vi "Link Control References.vi"(8 "error in (no error)":errorcluster, 10 "Control Map":T1[](array[typedef]), 11 "FunctionGenerator in":refnum<class "FunctionGenerator.lvclass">) -> (0 "error out":errorcluster, 3 "FunctionGenerator out":refnum<class "FunctionGenerator.lvclass">)   [LabVIEW 2019, in "FunctionGenerator.lvlib" / "FunctionGenerator.lvclass"]
uses:
  Library/FunctionGenerator.lvclass
  builds/Instruments/Instruments.lvlibp/Custom Controls/Control Element.ctl
  Library/FunctionGenerator.lvclass/FunctionGenerator.ctl
  builds/Instruments/Instruments.lvlibp/Library/Instruments.lvclass
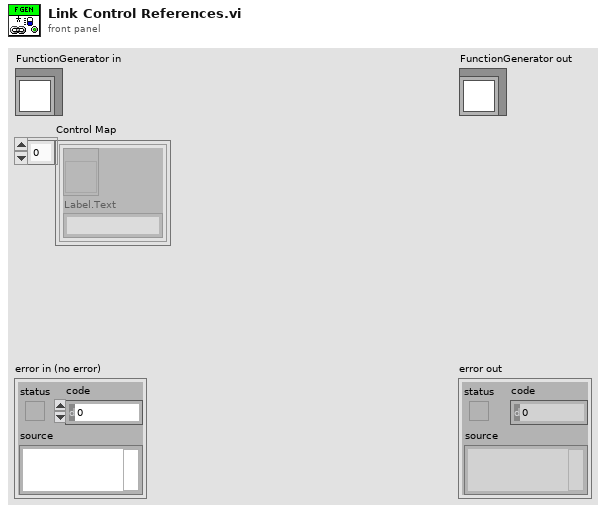
[diagram p1: front panel]
types:
  T1 = typedef "Instruments.lvlibp/Instruments.lvclass/Control Element.ctl" = cluster{refnum<vi>, "Label.Text":string}
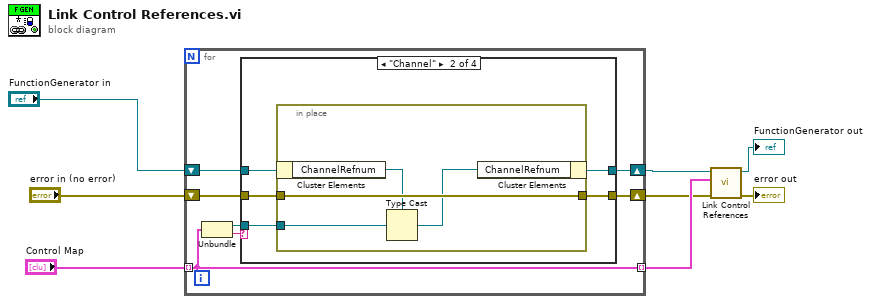
[diagram p0: block diagram]
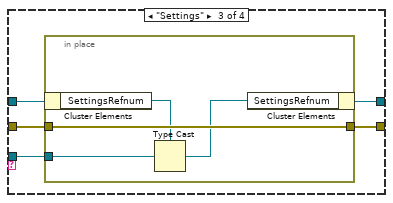
[diagram p3: hidden frame]
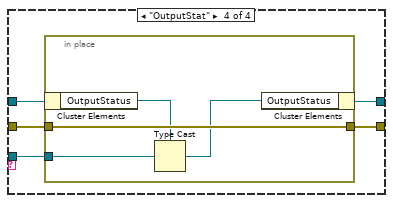
[diagram p4: hidden frame]
diagram:
  n1 = for {
    tunnel: "Control Map" -> [w13] mode=indexing
    tunnel: [w13] -> w5 mode=indexing
    shift-right: [w10] -> w3
    shift-left: "FunctionGenerator in" -> [w14]
    shift-right: [w9] -> w1
    shift-left: "error in (no error)" -> [w15]
    n2 = Unbundle(w13) -> (w11:refnum<vi>, "Label.Text"=w12:string)
    n3 = case shown="\"Channel\"" w12 {
      tunnel: w15 -> [w16 w20 w29 w38]
      tunnel: w14 -> [w17 w22 w31 w40]
      tunnel: w11 -> [_ w18 w27 w36]
      tunnel: [w17 w21 w30 w39] -> w10
      tunnel: [w16 w19 w28 w37] -> w9
      frame Default {
      }
      frame "Channel" {
        n4 = in-place {
          in-place-border: w20 -> [w26]
          in-place-border: [w26] -> w19
          in-place-border: w18 -> [w24]
          n5 = in-place-cluster #1(w22) -> ("ChannelRefnum"=w25:refnum<vi>)
          n6 = Type Cast(type=w25, x=w24) -> (*(type *) &x=w23:refnum<vi>)
          n7 = in-place-cluster #1("ChannelRefnum"=w23) -> (w21:refnum<class "FunctionGenerator.lvclass">)
        }
      }
      frame "Settings" {
        n8 = in-place {
          in-place-border: w29 -> [w35]
          in-place-border: [w35] -> w28
          in-place-border: w27 -> [w33]
          n9 = in-place-cluster #2(w31) -> ("SettingsRefnum"=w34:refnum<vi>)
          n10 = Type Cast(type=w34, x=w33) -> (*(type *) &x=w32:refnum<vi>)
          n11 = in-place-cluster #2("SettingsRefnum"=w32) -> (w30:refnum<class "FunctionGenerator.lvclass">)
        }
      }
      frame "OutputStat" {
        n12 = in-place {
          in-place-border: w38 -> [w44]
          in-place-border: [w44] -> w37
          in-place-border: w36 -> [w42]
          n13 = in-place-cluster #3(w40) -> ("OutputStatus"=w43:refnum<vi>)
          n14 = Type Cast(type=w43, x=w42) -> (*(type *) &x=w41:refnum<vi>)
          n15 = in-place-cluster #3("OutputStatus"=w41) -> (w39:refnum<class "FunctionGenerator.lvclass">)
        }
      }
    }
  }
  n16 = call-parent "Link Control References.vi"("error in (no error)"=w1, "Control Map"=w5, "Instruments in"=w3) -> ("error out"=→"error out":errorcluster, "Instruments out"=→"FunctionGenerator out":refnum<class "FunctionGenerator.lvclass">)  [unwired: 7 in]
